vi "IsSatisfied.vi"(10 "Product":refnum<class "Product.lvclass">, 11 "AndSpecification":refnum<class "AndSpecification.lvclass">) -> (2 "IsSatisfied":bool)   [LabVIEW 2018, in "AndSpecification.lvclass"]
uses:
  AndSpecification.lvclass
  Product/Product.lvclass
  AndSpecification.lvclass/AndSpecification.ctl
  IFilterSpecification/IFilterSpecification.lvclass
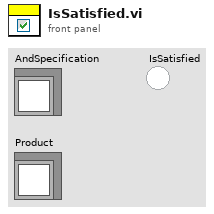
[diagram p1: front panel]
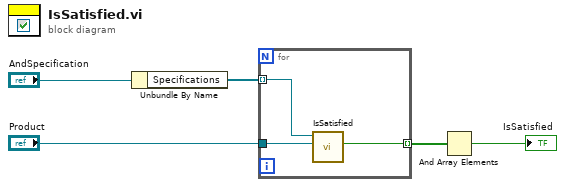
[diagram p0: block diagram]
diagram:
  n1 = Unbundle By Name("AndSpecification") -> ("Specifications"=w2:refnum<class "IFilterSpecification.lvclass">[])
  n2 = for {
    tunnel: [w6] -> w5 mode=indexing
    tunnel: "Product" -> [w7]
    tunnel: w2 -> [w8] mode=indexing
    n3 = call-dynamic "IsSatisfied.vi"("Product"=w7, "IFilterSpecification"=w8) -> ("IsSatisfied"=w6:bool)  [unwired: 9 in]
  }
  n4 = And Array Elements(Boolean array=w5) -> (logical AND=→"IsSatisfied":bool)
